vi "Actor.vi"(6 "Refs":refnum<class "Refs.lvclass">, 9 "Actor Ref":refnum<vi>, 10 "Spawn":refnum<class "Spawn.lvclass">, 11 "Actor in":refnum<class "Actor.lvclass">) -> (0 "Error out":errorcluster, 3 "Actor out":refnum<class "Actor.lvclass">)   [LabVIEW 2025, in "jettl.lvlib" / "Actor.lvclass"]
uses:
  Actor.lvclass
  Spawn/Spawn/Spawn.lvclass
  Refs/Refs.lvclass
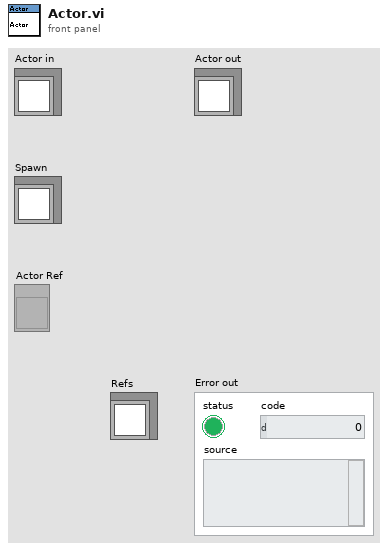
[diagram p1: front panel]
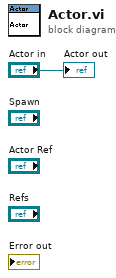
[diagram p0: block diagram]
diagram:
  "Actor out" <- "Actor in"
